vi "Handle Error.vi"(8 "error in (no error)":errorcluster, 11 "Rename in":refnum<class "Rename.lvclass">) -> (0 "error out":errorcluster, 2 "Stop Module":bool, 3 "Rename out":refnum<class "Rename.lvclass">)   [LabVIEW 2015, in "Generic Module Library.lvlib" / "Template G_Module.lvlib"]
uses:
  Template G_Module.lvlib
  Module Class/Rename.lvclass
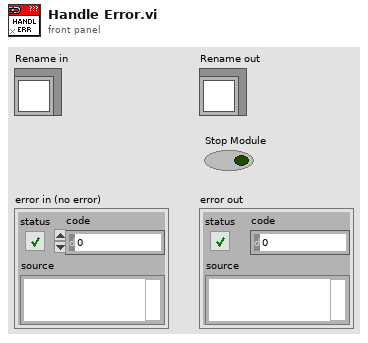
[diagram p1: front panel]
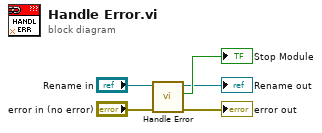
[diagram p0: block diagram]
diagram:
  n1 = call-dynamic "Handle Error.vi"("error in (no error)"="error in (no error)", "Module Data In"="Rename in") -> ("error out"=→"error out":errorcluster, "Stop Module"=→"Stop Module":bool, "Module Data Out"=→"Rename out":refnum<class "Rename.lvclass">)  [unwired: 7 in]
